vi "Initialize.vi"(6 "TTL Lines":T1, 8 "error in (no error)":errorcluster, 9 "TTL":refnum<class "TTL.lvclass">, 10 "Pressure Control Config":T2, 11 "Pressure Control in":refnum<class "Pressure Control.lvclass">) -> (0 "error out":errorcluster, 3 "Pressure Control out":refnum<class "Pressure Control.lvclass">)   [LabVIEW 2011, in "Pressure Control.lvclass"]
uses:
  Pressure Control.lvclass
  Pressure Control Config.ctl
  TTL/TTL.lvclass
  TTL/TTL Lines.ctl
  Pressure Control Status Data.ctl
  Pressure Control.lvclass/Pressure Control.ctl
  <vilib>/DAQmx/create/channels.llb/DAQmx Create Channel (AI-Voltage-Basic).vi
  C:/Program Files/National Instruments/LabVIEW 2011/resource/objmgr/daqmx.rc
panel:
  out "AI.TermCfg":i32(ring)=10083 items=["RSE"=10083, "NRSE"=10078, "Differential"=10106, "Pseudodifferential"=12529]
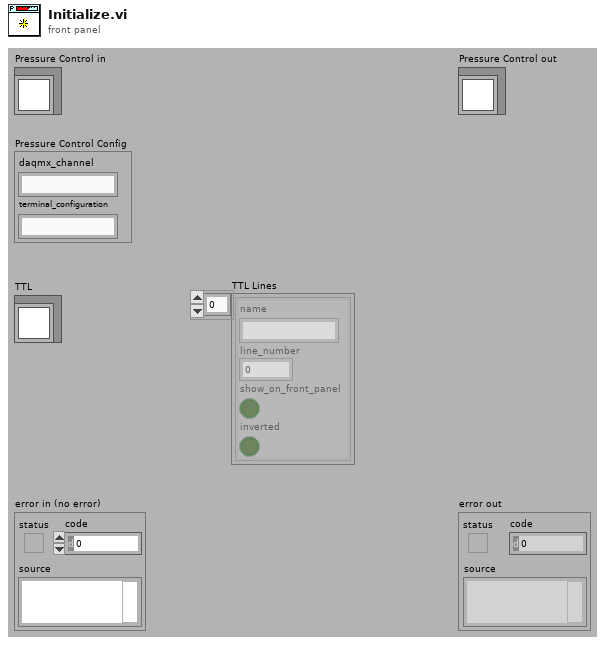
[diagram p1: front panel]
types:
  T1 = typedef "TTL Lines.ctl" = cluster{"name":string, "line_number":u8, "show_on_front_panel":bool, "inverted":bool}[]
  T2 = typedef "Pressure Control.lvclass/Pressure Control Config.ctl" = cluster{"daqmx_channel":string, "terminal_configuration":string}
  T3 = typedef "Pressure Control.lvclass/Pressure Control Status Data.ctl" = cluster{"Zero pressure level":dbl}
  T4 = typedef "LVStringsAndValuesArrayTypeDef.ctl" = cluster{"String":string, "Value":i32}[]
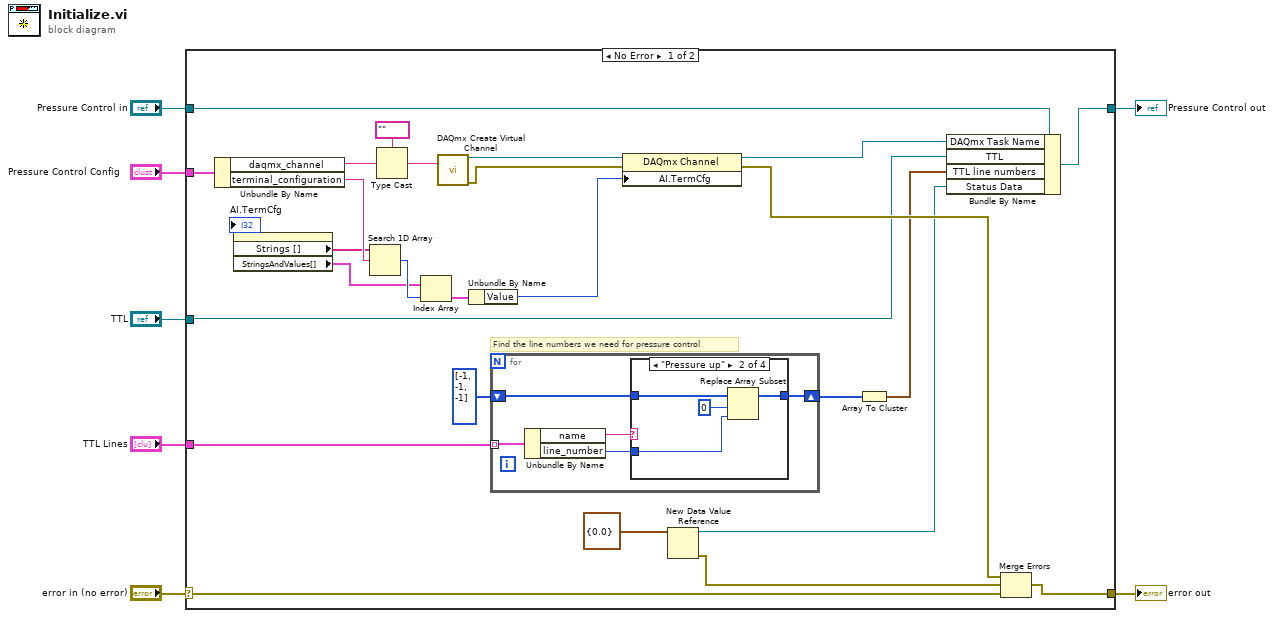
[diagram p0: block diagram]
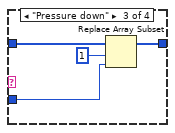
[diagram p3: hidden frame]
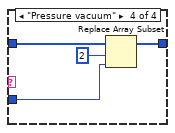
[diagram p4: hidden frame]
diagram:
  n1 = case shown="No Error" "error in (no error)" {
    selector: "error in (no error)" -> [w23 w53]
    tunnel: [w22 w53] -> w6
    tunnel: [w30 w52] -> w4
    tunnel: "Pressure Control in" -> [w32 w52]
    tunnel: "Pressure Control Config" -> [w16 _]
    tunnel: "TTL" -> [w29 _]
    tunnel: "TTL Lines" -> [w28 _]
    frame No Error {
      # "Find the line numbers we need for pressure control"
      n2 = Unbundle By Name(w16) -> ("daqmx_channel"=w15:string, "terminal_configuration"=w13:string)
      n3 = property on="AI.TermCfg" class="Ring (strict)"() -> ("Strings []"=w12:string[], "StringsAndValues[]"=w10:T4)  [unwired: 2 in, 2 out]
      n4 = Search 1D Array(1D array=w12, element=w13) -> (index of element=w11:i32)  [unwired: 1 in]
      n5 = Type Cast(type=tag "" ("DAQmx Physical Channel"), x=w15) -> (*(type *) &x=w14:tag)
      n6 = Index Array(array=w10, index=w11) -> (element=w9:cluster{"String":string, "Value":i32})
      n7 = call-poly <vilib>:"DAQmx Create Virtual Channel.vi"("physical channels"=w14) -> ("task out"=w31:refnum<k21>, "error out"=w18:errorcluster)  [unwired: 13 in]
      n8 = Unbundle By Name(w9) -> ("Value"=w8:i32)
      n9 = for {
        tunnel: w28 -> [w38] mode=indexing
        shift-right: [w35] -> w26
        shift-left: i32[] [-1, -1, -1] -> [w36]
        n10 = Unbundle By Name(w38) -> ("name"=w37:string, "line_number"=w34:u8)
        n11 = case shown="\"Pressure up\"" w37 {
          tunnel: w36 -> [w39 w43 w47 w51]
          tunnel: [w39 w42 w46 w50] -> w35
          tunnel: w34 -> [_ w40 w44 w48]
          frame Default {
          }
          frame "Pressure up" {
            n12 = Replace Array Subset(array=w43, new element=w40, index=0) -> (w42:i32[])
          }
          frame "Pressure down" {
            n13 = Replace Array Subset(array=w47, new element=w44, index=1) -> (w46:i32[])
          }
          frame "Pressure vacuum" {
            n14 = Replace Array Subset(array=w51, new element=w48, index=2) -> (w50:i32[])
          }
        }
      }
      n15 = property class="DAQmx Channel"(reference=w31, error in=w18, "AI.TermCfg"=w8) -> (reference out=w19:refnum<k21>, error out=w33:errorcluster)
      n16 = New Data Value Reference(data value=T3 {"Zero pressure level"=0.0} ("Pressure Control Status Data")) -> (data value reference=w20:refnum<data-value>, error out=w21:errorcluster)  [unwired: 1 in]
      n17 = Array To Cluster(array=w26) -> (cluster=w25:cluster{"[0]":i32, "[1]":i32, "[2]":i32})
      n18 = Bundle By Name(cluster=w32, "DAQmx Task Name"=w19, "TTL"=w29, "TTL line numbers"=w25, "Status Data"=w20) -> (w30:refnum<class "Pressure Control.lvclass">)
      n19 = Merge Errors(w33, w21, w23) -> (w22:errorcluster)
    }
    frame Error {
    }
  }
  "error out" <- w6
  "Pressure Control out" <- w4
